vi "Func-엑셀 데이터를 그래프로 출력.vi"() -> ()   [LabVIEW 2015] (continued)
-10.012\n-18.3\t-18.31\t-10.011\n-18.3\t-18.31\t-10.009\n-18.3\t-18.31\t-10.008\n-18.3\t-18.31\t-10.009\n-18.3\t-18.31\t-10.009\n-18.3\t-18.31\t-10.008\n-18.3\t-18.31\t-10.003\n-18.3\t-18.31\t-10.002\n-18.3\t-18.31\t-10\n-18.3\t-18.31\t-10.001\n-18.3\t-18.31\t-10\n-18.3\t-18.31\t-9.994\n-18.3\t-18.31\t-9.993\n-18.3\t-18.31\t-9.993\n-18.3\t-18.31\t-9.993\n-18.3\t-18.31\t-9.989\n-18.3\t-18.31\t-9.99\n-18.3\t-18.31\t-9.995\n-18.3\t-18.31\t-9.995\n-18.3\t-18.31\t-9.993\n-18.3\t-18.31\t-9.99\n-18.3\t-18.31\t-9.987\n-18.3\t-18.31\t-9.984\n-18.3\t-18.31\t-9.979\n-18.3\t-18.31\t-9.975\n-18.3\t-18.31\t-9.972\n-18.3\t-18.31\t-9.973\n-18.3\t-18.31\t-9.969\n-18.3\t-18.31\t-9.965\n-18.3\t-18.31\t-9.962\n-18.3\t-18.31\t-9.963\n-18.3\t-18.31\t-9.964\n-18.3\t-18.31\t-9.962\n-18.3\t-18.31\t-9.967\n-18.3\t-18.31\t-9.969\n-18.3\t-18.31\t-9.97\n-18.3\t-18.31\t-9.971\n-18.3\t-18.31\t-9.968\n-18.3\t-18.31\t-9.967\n-18.3\t-18.31\t-9.961\n-18.3\t-18.31\t-9.957\n-18.3\t-18.31\t-9.955\n-18.3\t-18.31\t-9.948\n-18.3\t-18.31\t-9.948\n-18.3\t-18.31\t-9.945\n-18.3\t-18.31\t-9.948\n-18.3\t-18.31\t-9.948\n-18.3\t-18.31\t-9.948\n-18.3\t-18.31\t-9.95\n-18.3\t-18.31\t-9.949\n-18.3\t-18.31\t-9.947\n-18.3\t-18.31\t-9.941\n-18.3\t-18.31\t-9.941\n-18.3\t-18.31\t-9.939\n-18.3\t-18.31\t-9.937\n-18.3\t-18.31\t-9.936\n-18.3\t-18.31\t-9.938\n-18.3\t-18.31\t-9.933\n-18.3\t-18.31\t-9.931\n-18.3\t-18.31\t-9.929\n-18.3\t-18.31\t-9.925\n-18.3\t-18.31\t-9.925\n-18.3\t-18.31\t-9.925\n-18.3\t-18.31\t-9.927\n-18.3\t-18.31\t-9.927\n-18.3\t-18.31\t-9.93\n-18.3\t-18.31\t-9.926\n-18.3\t-18.31\t-9.923\n-18.3\t-18.31\t-9.92\n-18.3\t-18.31\t-9.916\n-18.3\t-18.31\t-9.915\n-18.3\t-18.31\t-9.911\n-18.3\t-18.31\t-9.911\n-18.3\t-18.31\t-9.911\n-18.3\t-18.31\t-9.91\n-18.3\t-18.31\t-9.911\n-18.3\t-18.31\t-9.912\n-18.3\t-18.31\t-9.911\n-18.3\t-18.31\t-9.911\n-18.3\t-18.31\t-9.908\n-18.3\t-18.31\t-9.909\n-18.3\t-18.31\t-9.905\n-18.3\t-18.31\t-9.902\n-18.3\t-18.31\t-9.899\n-18.3\t-18.31\t-9.898\n-18.3\t-18.31\t-9.895\n-18.3\t-18.31\t-9.894\n-18.3\t-18.31\t-9.895\n-18.3\t-18.31\t-9.891\n-18.3\t-18.31\t-9.886\n-18.3\t-18.31\t-9.886\n-18.3\t-18.31\t-9.885\n-18.3\t-18.31\t-9.882\n-18.3\t-18.31\t-9.877\n-18.3\t-18.31\t-9.878\n-18.3\t-18.31\t-9.88\n-18.3\t-18.31\t-9.879\n-18.3\t-18.31\t-9.879\n-18.3\t-18.31\t-9.879\n-18.3\t-18.31\t-9.879\n-18.3\t-18.31\t-9.875\n-18.3\t-18.31\t-9.875\n-18.3\t-18.31\t-9.875\n-18.3\t-18.31\t-9.873\n-18.3\t-18.31\t-9.87\n-18.3\t-18.31\t-9.868\n-18.3\t-18.31\t-9.868\n-18.3\t-18.31\t-9.867\n-18.3\t-18.31\t-9.865\n-18.3\t-18.31\t-9.864\n-18.3\t-18.31\t-9.864\n-18.3\t-18.31\t-9.866\n-18.3\t-18.31\t-9.865\n-18.3\t-18.31\t-9.863\n-18.3\t-18.31\t-9.861\n-18.3\t-18.31\t-9.861\n-18.3\t-18.31\t-9.866\n-18.3\t-18.31\t-9.861\n-18.3\t-18.31\t-9.861\n-18.3\t-18.31\t-9.86\n-18.3\t-18.31\t-9.856\n-18.3\t-18.31\t-9.852\n-18.3\t-18.31\t-9.849\n-18.3\t-18.31\t-9.847\n-18.3\t-18.31\t-9.844\n-18.3\t-18.31\t-9.842\n-18.3\t-18.31\t-9.844\n-18.3\t-18.31\t-9.846\n-18.3\t-18.31\t-9.841\n-18.3\t-18.31\t-9.84\n-18.3\t-18.31\t-9.84\n-18.3\t-18.31\t-9.841\n-18.3\t-18.31\t-9.837\n-18.3\t-18.31\t-9.835\n-18.3\t-18.31\t-9.836\n-18.3\t-18.31\t-9.834\n-18.3\t-18.31\t-9.834\n-18.3\t-18.31\t-9.832\n-18.3\t-18.31\t-9.832\n-18.3\t-18.31\t-9.832\n-18.3\t-18.31\t-9.83\n-18.3\t-18.31\t-9.833\n-18.3\t-18.31\t-9.83\n-18.3\t-18.31\t-9.827\n-18.3\t-18.31\t-9.824\n-18.3\t-18.31\t-9.823\n-18.3\t-18.31\t-9.823\n-18.3\t-18.31\t-9.82\n-18.3\t-18.31\t-9.82\n-18.3\t-18.31\t-9.821\n-18.3\t-18.31\t-9.82\n-18.3\t-18.31\t-9.821\n-18.3\t-18.31\t-9.821\n-18.3\t-18.31\t-9.821\n-18.3\t-18.31\t-9.822\n-18.3\t-18.31\t-9.82\n-18.3\t-18.31\t-9.817\n-18.3\t-18.31\t-9.815\n-18.3\t-18.31\t-9.812\n-18.3\t-18.31\t-9.807\n-18.3\t-18.31\t-9.801\n-18.3\t-18.31\t-9.803\n-18.3\t-18.31\t-9.802\n-18.3\t-18.31\t-9.802\n-18.3\t-18.31\t-9.801\n-18.3\t-18.31\t-9.8\n-18.3\t-18.31\t-9.799\n-18.3\t-18.31\t-9.799\n-18.3\t-18.31\t-9.797\n-18.3\t-18.31\t-9.797\n-18.3\t-18.31\t-9.795\n-18.3\t-18.31\t-9.795\n-18.3\t-18.31\t-9.793\n-18.3\t-18.31\t-9.788\n-18.3\t-18.31\t-9.79\n-18.3\t-18.31\t-9.788\n-18.3\t-18.31\t-9.789\n-18.3\t-18.31\t-9.785\n-18.3\t-18.31\t-9.787\n-18.3\t-18.31\t-9.786\n-18.3\t-18.31\t-9.784\n-18.3\t-18.31\t-9.782\n-18.3\t-18.31\t-9.782\n-18.3\t-18.31\t-9.782\n-18.3\t-18.31\t-9.783\n-18.3\t-18.31\t-9.783\n-18.3\t-18.31\t-9.774\n-18.3\t-18.31\t-9.775\n-18.3\t-18.31\t-9.77\n-18.3\t-18.31\t-9.769\n-18.3\t-18.31\t-9.768\n-18.3\t-18.31\t-9.769\n-18.3\t-18.31\t-9.778\n-18.3\t-18.31\t-9.775\n-18.3\t-18.31\t-9.779\n-18.3\t-18.31\t-9.777\n-18.3\t-18.31\t-9.777\n-18.3\t-18.31\t-9.778\n-18.3\t-18.31\t-9.77\n-18.3\t-18.31\t-9.767\n-18.3\t-18.31\t-9.765\n-18.3\t-18.31\t-9.76\n-18.3\t-18.31\t-9.755\n-18.3\t-18.31\t-9.75\n-18.3\t-18.31\t-9.749\n-18.3\t-18.31\t-9.749\n-18.3\t-18.31\t-9.748\n-18.3\t-18.31\t-9.751\n-18.3\t-18.31\t-9.752\n-18.3\t-18.31\t-9.754\n-18.3\t-18.31\t-9.752\n-18.3\t-18.31\t-9.752\n-18.3\t-18.31\t-9.748\n-18.3\t-18.31\t-9.745\n-18.3\t-18.31\t-9.743\n-18.3\t-18.31\t-9.739\n-18.3\t-18.31\t-9.74\n-18.3\t-18.31\t-9.74\n-18.3\t-18.31\t-9.74\n-18.3\t-18.31\t-9.735\n-18.3\t-18.31\t-9.735\n-18.3\t-18.31\t-9.736\n-18.3\t-18.31\t-9.734\n-18.3\t-18.31\t-9.73\n-18.3\t-18.31\t-9.732\n-18.3\t-18.31\t-9.736\n-18.3\t-18.31\t-9.733\n-18.3\t-18.31\t-9.732\n-18.3\t-18.31\t-9.729\n-18.3\t-18.31\t-9.729\n-18.3\t-18.31\t-9.725\n-18.3\t-18.31\t-9.72\n-18.3\t-18.31\t-9.721\n-18.3\t-18.31\t-9.72\n-18.3\t-18.31\t-9.722\n-18.3\t-18.31\t-9.722\n-18.3\t-18.31\t-9.721\n-18.3\t-18.31\t-9.722\n-18.3\t-18.31\t-9.721\n-18.3\t-18.31\t-9.721\n-18.3\t-18.31\t-9.718\n-18.3\t-18.31\t-9.719\n-18.3\t-18.31\t-9.718\n-18.3\t-18.31\t-9.719\n-18.3\t-18.31\t-9.721\n-18.3\t-18.31\t-9.719\n-18.3\t-18.31\t-9.716\n-18.3\t-18.31\t-9.711\n-18.3\t-18.31\t-9.712\n-18.3\t-18.31\t-9.712\n-18.3\t-18.31\t-9.707\n-18.3\t-18.31\t-9.708\n-18.3\t-18.31\t-9.71\n-18.3\t-18.31\t-9.709\n-18.3\t-18.31\t-9.705\n-18.3\t-18.31\t-9.704\n-18.3\t-18.31\t-9.702\n-18.3\t-18.31\t-9.7\n-18.3\t-18.31\t-9.7\n-18.3\t-18.31\t-9.702\n-18.3\t-18.31\t-9.704\n-18.3\t-18.31\t-9.701\n-18.3\t-18.31\t-9.702\n-18.3\t-18.31\t-9.699\n-18.3\t-18.31\t-9.698\n-18.3\t-18.31\t-9.695\n-18.3\t-18.31\t-9.695\n-18.3\t-18.31\t-9.695\n-18.3\t-18.31\t-9.694\n-18.3\t-18.31\t-9.695\n-18.3\t-18.31\t-9.691\n-18.3\t-18.31\t-9.689\n-18.3\t-18.31\t-9.686\n-18.3\t-18.31\t-9.684\n-18.3\t-18.31\t-9.68\n-18.3\t-18.31\t-9.678\n-18.3\t-18.31\t-9.679\n-18.3\t-18.31\t-9.68\n-18.3\t-18.31\t-9.68\n-18.3\t-18.31\t-9.678\n-18.3\t-18.31\t-9.68\n-18.3\t-18.31\t-9.679\n-18.3\t-18.31\t-9.677\n-18.3\t-18.31\t-9.675\n-18.3\t-18.31\t-9.673\n-18.3\t-18.31\t-9.674\n-18.3\t-18.31\t-9.675\n-18.3\t-18.31\t-9.674\n-18.3\t-18.31\t-9.672\n-18.3\t-18.31\t-9.67\n-18.3\t-18.31\t-9.67\n-18.3\t-18.31\t-9.669\n-18.3\t-18.31\t-9.666\n-18.3\t-18.31\t-9.667\n-18.3\t-18.31\t-9.666\n-18.3\t-18.31\t-9.666\n-18.3\t-18.31\t-9.664\n-18.3\t-18.31\t-9.663\n-18.3\t-18.31\t-9.663\n-18.3\t-18.31\t-9.663\n-18.3\t-18.31\t-9.661\n-18.3\t-18.31\t-9.656\n-18.3\t-18.31\t-9.654\n-18.3\t-18.31\t-9.654\n-18.3\t-18.31\t-9.654\n-18.3\t-18.31\t-9.652\n-18.3\t-18.31\t-9.65\n-18.3\t-18.31\t-9.652\n-18.3\t-18.31\t-9.654\n-18.3\t-18.31\t-9.65\n-18.3\t-18.31\t-9.647\n-18.3\t-18.31\t-9.644\n-18.3\t-18.31\t-9.646\n-18.3\t-18.31\t-9.646\n-18.3\t-18.31\t-9.642\n-18.3\t-18.31\t-9.645\n-18.3\t-18.31\t-9.643\n-18.3\t-18.31\t-9.645\n-18.3\t-18.31\t-9.639\n-18.3\t-18.31\t-9.639\n-18.3\t-18.31\t-9.639\n-18.3\t-18.31\t-9.639\n-18.3\t-18.31\t-9.641\n-18.3\t-18.31\t-9.637\n-18.3\t-18.31\t-9.639\n-18.3\t-18.31\t-9.639\n-18.3\t-18.31\t-9.637\n-18.3\t-18.31\t-9.629\n-18.3\t-18.31\t-9.624\n-18.3\t-18.31\t-9.622\n-18.3\t-18.31\t-9.62\n-18.3\t-18.31\t-9.619\n-18.3\t-18.31\t-9.62\n-18.3\t-18.31\t-9.62\n-18.3\t-18.31\t-9.62\n-18.3\t-18.31\t-9.621\n-18.3\t-18.31\t-9.624\n-18.3\t-18.31\t-9.625\n-18.3\t-18.31\t-9.622\n-18.3\t-18.31\t-9.625\n-18.3\t-18.31\t-9.624\n-18.3\t-18.31\t-9.621\n-18.3\t-18.31\t-9.619\n-18.3\t-18.31\t-9.613\n-18.3\t-18.31\t-9.609\n-18.3\t-18.31\t-9.607\n-18.3\t-18.31\t-9.607\n-18.3\t-18.31\t-9.605\n-18.3\t-18.31\t-9.609\n-18.3\t-18.31\t-9.613\n-18.3\t-18.31\t-9.613\n-18.3\t-18.31\t-9.614\n-18.3\t-18.31\t-9.613\n-18.3\t-18.31\t-9.611\n-18.3\t-18.31\t-9.607\n-18.3\t-18.31\t-9.604\n-18.3\t-18.31\t-9.604\n-18.3\t-18.31\t-9.601\n-18.3\t-18.31\t-9.6\n-18.3\t-18.31\t-9.602\n-18.3\t-18.31\t-9.604\n-18.3\t-18.31\t-9.603\n-18.3\t-18.31\t-9.602\n-18.3\t-18.31\t-9.603\n-18.3\t-18.31\t-9.606\n-18.3\t-18.31\t-9.604\n-18.3\t-18.31\t-9.6\n-18.3\t-18.31\t-9.602\n-18.3\t-18.31\t-9.6\n-18.3\t-18.31\t-9.601\n-18.3\t-18.31\t-9.598\n-18.3\t-18.31\t-9.598\n-18.3\t-18.31\t-9.595\n-18.3\t-18.31\t-9.593\n-18.3\t-18.31\t-9.594\n-18.3\t-18.31\t-9.594\n-18.3\t-18.31\t-9.595\n-18.3\t-18.31\t-9.592\n-18.3\t-18.31\t-9.598\n-18.3\t-18.31\t-9.596\n-18.3\t-18.31\t-9.594\n-18.3\t-18.31\t-9.588\n-18.3\t-18.31\t-9.587\n-18.3\t-18.31\t-9.585\n-18.3\t-18.31\t-9.579\n-18.3\t-18.31\t-9.579\n-18.3\t-18.31\t-9.574\n-18.3\t-18.31\t-9.578\n-18.3\t-18.31\t-9.575\n-18.3\t-18.31\t-9.575\n-18.3\t-18.31\t-9.575\n-18.3\t-18.31\t-9.573\n-18.227\t-18.25\t-9.109\n-18.143\t-18.18\t-9.102\n-18.06\t-18.12\t-9.09\n-17.977\t-18.32\t-9.09\n-17.893\t-18.38\t-9.096\n-17.81\t-18.43\t-9.092\n-17.727\t-18.51\t-9.087\n-17.643\t-18.57\t-9.085\n-17.56\t-18.62\t-9.089\n-17.477\t-18.68\t-9.081\n-17.393\t-18.74\t-9.075\n-17.31\t-18.79\t-9.079\n-17.227\t-18.83\t-9.069\n-17.143\t-18.86\t-9.073\n-17.06\t-18.88\t-9.07\n-16.977\t-18.89\t-9.072\n-16.893\t-18.87\t-9.071\n-16.81\t-18.86\t-9.067\n-16.727\t-18.84\t-9.071\n-16.643\t-18.82\t-9.076\n-16.56\t-18.78\t-9.072\n-16.477\t-18.73\t-9.069\n-16.393\t-18.67\t-9.07\n-16.31\t-18.62\t-9.075\n-16.227\t-18.55\t-9.071\n-16.143\t-18.48\t-9.073\n-16.06\t-18.41\t-9.074\n-15.977\t-18.34\t-9.069\n-15.893\t-18.27\t-9.074\n-15.81\t-18.18\t-9.077\n-15.727\t-18.1\t-9.073\n-15.643\t-18.01\t-9.086\n-15.56\t-17.91\t-9.08\n-15.477\t-17.82\t-9.078\n-15.393\t-17.73\t-9.079\n-15.31\t-17.63\t-9.077\n-15.227\t-17.55\t-9.076\n-15.143\t-17.46\t-9.087\n-15.06\t-17.36\t-9.075\n-14.977\t-17.27\t-9.072\n-14.893\t-17.17\t-9.07\n-14.81\t-17.08\t-9.071\n-14.727\t-16.99\t-9.069\n-14.643\t-16.9\t-9.069\n-14.56\t-16.81\t-9.06\n-14.477\t-16.73\t-9.06\n-14.393\t-16.65\t-9.052\n-14.31\t-16.57\t-9.044\n-14.227\t-16.48\t-9.036\n-14.143\t-16.4\t-9.035\n-14.06\t-16.31\t-9.027\n-13.977\t-16.23\t-9.016\n-13.893\t-16.16\t-9.013\n-13.81\t-16.07\t-9\n-13.727\t-15.99\t-8.993\n-13.643\t-15.92\t-8.982\n-13.56\t-15.85\t-8.973\n-13.477\t-15.77\t-8.961\n-13.393\t-15.69\t-8.946\n-13.31\t-15.61\t-8.935\n-13.227\t-15.53\t-8.924\n-13.143\t-15.45\t-8.911\n-13.06\t-15.38\t-8.898\n-12.977\t-15.3\t-8.889\n-12.893\t-15.23\t-8.865\n-12.81\t-15.14\t-8.849\n-12.727\t-15.08\t-8.828\n-12.643\t-15\t-8.819\n-12.56\t-14.92\t-8.789\n-12.477\t-14.84\t-8.776\n-12.393\t-14.76\t-8.756\n-12.31\t-14.68\t-8.729\n-12.227\t-14.61\t-8.712\n-12.143\t-14.54\t-8.686\n-12.06\t-14.46\t-8.679\n-11.977\t-14.39\t-8.652\n-11.893\t-14.31\t-8.623\n-11.81\t-14.24\t-8.606\n-11.727\t-14.15\t-8.582\n-11.643\t-14.07\t-8.555\n-11.56\t-13.99\t-8.529\n-11.477\t-13.91\t-8.505\n-11.393\t-13.83\t-8.469\n-11.31\t-13.75\t-8.455\n-11.227\t-13.67\t-8.418\n-11.143\t-13.59\t-8.395\n-11.06\t-13.51\t-8.368\n-10.977\t-13.43\t-8.341\n-10.893\t-13.35\t-8.308\n-10.81\t-13.27\t-8.281\n-10.727\t-13.19\t-8.244\n-10.643\t-13.11\t-8.217\n-10.56\t-13.04\t-8.188\n-10.477\t-12.96\t-8.153\n-10.393\t-12.89\t-8.131\n-10.31\t-12.81\t-8.098\n-10.227\t-12.74\t-8.061\n-10.143\t-12.66\t-8.029\n-10.06\t-12.6\t-8.002\n-9.977\t-12.52\t-7.962\n-9.893\t-12.44\t-7.935\n-9.81\t-12.36\t-7.898\n-9.727\t-12.28\t-7.868\n-9.643\t-12.21\t-7.835\n-9.56\t-12.12\t-7.791\n-9.477\t-12.05\t-7.763\n-9.393\t-11.96\t-7.726\n-9.31\t-11.88\t-7.688\n-9.227\t-11.8\t-7.656\n-9.143\t-11.74\t-7.614\n-9.06\t-11.65\t-7.577\n-8.977\t-11.57\t-7.539\n-8.893\t-11.5\t-7.497\n-8.81\t-11.42\t-7.463\n-8.727\t-11.34\t-7.415\n-8.643\t-11.26\t-7.379\n-8.56\t-11.19\t-7.333\n-8.477\t-11.11\t-7.288\n-8.393\t-11.03\t-7.259\n-8.31\t-10.94\t-7.211\n-8.227\t-10.86\t-7.166\n-8.143\t-10.78\t-7.121\n-8.06\t-10.7\t-7.076\n-7.977\t-10.62\t-7.039\n-7.893\t-10.53\t-6.994\n-7.81\t-10.45\t-6.95\n-7.727\t-10.37\t-6.907\n-7.643\t-10.28\t-6.863\n-7.56\t-10.2\t-6.817\n-7.477\t-10.12\t-6.769\n-7.393\t-10.03\t-6.723\n-7.31\t-9.95\t-6.679\n-7.227\t-9.87\t-6.632\n-7.143\t-9.79\t-6.595\n-7.06\t-9.72\t-6.54\n-6.977\t-9.65\t-6.496\n-6.893\t-9.57\t-6.446\n-6.81\t-9.5\t-6.399\n-6.727\t-9.41\t-6.343\n-6.643\t-9.34\t-6.3\n-6.56\t-9.26\t-6.254\n-6.477\t-9.18\t-6.203\n-6.393\t-9.1\t-6.157\n-6.31\t-9.03\t-6.098\n-6.227\t-8.95\t-6.05\n-6.143\t-8.87\t-6.001\n-6.06\t-8.79\t-5.95\n-5.977\t-8.71\t-5.889\n-5.893\t-8.63\t-5.837\n-5.81\t-8.55\t-5.788\n-5.727\t-8.48\t-5.736\n-5.643\t-8.4\t-5.683\n-5.56\t-8.32\t-5.622\n-5.477\t-8.24\t-5.575\n-5.393\t-8.17\t-5.516\n-5.31\t-8.08\t-5.458\n-5.227\t-8\t-5.407\n-5.143\t-7.92\t-5.352\n-5.06\t-7.84\t-5.297\n-4.977\t-7.76\t-5.236\n-4.893\t-7.69\t-5.187\n-4.81\t-7.6\t-5.127\n-4.727\t-7.53\t-5.066\n-4.643\t-7.45\t-5.014\n-4.56\t-7.36\t-4.957\n-4.477\t-7.28\t-4.905\n-4.393\t-7.21\t-4.846\n-4.31\t-7.13\t-4.779\n-4.227\t-7.04\t-4.722\n-4.143\t-6.96\t-4.671\n-4.06\t-6.87\t-4.606\n-3.977\t-6.79\t-4.545\n-3.893\t-6.71\t-4.485\n-3.81\t-6.64\t-4.427\n-3.727\t-6.56\t-4.373\n-3.643\t-6.47\t-4.308\n-3.56\t-6.4\t-4.246\n-3.477\t-6.32\t-4.18\n-3.393\t-6.24\t-4.129\n-3.31\t-6.17\t-4.067\n-3.227\t-6.08\t-4.008\n-3.143\t-6\t-3.941\n-3.06\t-5.92\t-3.88\n-2.977\t-5.84\t-3.825\n-2.893\t-5.76\t-3.755\n-2.81\t-5.69\t-3.699\n-2.727\t-5.6\t-3.637\n-2.643\t-5.52\t-3.577\n-2.56\t-5.44\t-3.504\n-2.477\t-5.36\t-3.445\n-2.393\t-5.28\t-3.382\n-2.31\t-5.2\t-3.318\n-2.227\t-5.12\t-3.262\n-2.143\t-5.05\t-3.192\n-2.06\t-4.97\t-3.136\n-1.977\t-4.89\t-3.071\n-1.893\t-4.81\t-3.002\n-1.81\t-4.72\t-2.941\n-1.727\t-4.63\t-2.881\n-1.643\t-4.55\t-2.809\n-1.56\t-4.46\t-2.746\n-1.477\t-4.39\t-2.687\n-1.393\t-4.31\t-2.615\n-1.31\t-4.22\t-2.555\n-1.227\t-4.14\t-2.477\n-1.143\t-4.06\t-2.428\n-1.06\t-3.99\t-2.352\n-0.977\t-3.9\t-2.289\n-0.893\t-3.8\t-2.217\n-0.81\t-3.72\t-2.159\n-0.727\t-3.64\t-2.092\n-0.643\t-3.56\t-2.022\n-0.56\t-3.48\t-1.96\n-0.477\t-3.41\t-1.9\n-0.393\t-3.32\t-1.831\n-0.31\t-3.25\t-1.765\n-0.227\t-3.17\t-1.698\n-0.143\t-3.09\t-1.629\n-0.06\t-3\t-1.562\n0.023\t-2.93\t-1.496\n0.107\t-2.85\t-1.419\n0.19\t-2.77\t-1.354\n0.273\t-2.7\t-1.29\n0.357\t-2.61\t-1.221\n0.44\t-2.53\t-1.153\n0.523\t-2.45\t-1.084\n0.607\t-2.37\t-1.016\n0.69\t-2.29\t-0.95\n0.773\t-2.22\t-0.875\n0.857\t-2.14\t-0.811\n0.94\t-2.06\t-0.741\n1.023\t-1.99\t-0.668\n1.107\t-1.91\t-0.607\n1.19\t-1.84\t-0.53\n1.273\t-1.75\t-0.467\n1.357\t-1.68\t-0.404\n1.44\t-1.59\t-0.325\n1.523\t-1.51\t-0.259\n1.607\t-1.44\t-0.194\n1.69\t-1.35\t-0.114\n1.773\t-1.27\t-0.052\n1.857\t-1.2\t0.02\n1.94\t-1.12\t0.099\n2.023\t-1.04\t0.156\n2.107\t-0.96\t0.223\n2.19\t-0.88\t0.305\n2.273\t-0.8\t0.365\n2.357\t-0.72\t0.436\n2.44\t-0.64\t0.509\n2.523\t-0.56\t0.589\n2.607\t-0.48\t0.65\n2.69\t-0.41\t0.719\n2.773\t-0.33\t0.798\n2.857\t-0.25\t0.863\n2.94\t-0.16\t0.939\n3.023\t-0.08\t1.005\n3.107\t0\t1.065\n3.19\t0.08\t1.145\n3.3\t0.14\t1.216\n3.3\t0.15\t1.219\n3.3\t0.16\t1.222\n3.3\t0.18\t1.229\n3.3\t0.18\t1.238\n3.3\t0.19\t1.246\n3.3\t0.2\t1.252\n3.3\t0.21\t1.26\n3.3\t0.22\t1.266\n3.3\t0.23\t1.275\n3.3\t0.23\t1.279\n3.3\t0.25\t1.286\n3.3\t0.25\t1.295\n3.3\t0.25\t1.304\n3.3\t0.26\t1.311\n3.3\t0.27\t1.316\n3.3\t0.28\t1.327\n3.3\t0.29\t1.33\n3.3\t0.29\t1.333\n3.3\t0.3\t1.335\n3.3\t0.31\t1.337\n3.3\t0.32\t1.343\n3.3\t0.33\t1.349\n3.3\t0.34\t1.358\n3.3\t0.35\t1.369\n3.3\t0.35\t1.378\n3.3\t0.36\t1.387\n3.3\t0.37\t1.401\n3.3\t0.38\t1.41\n3.3\t0.39\t1.414\n3.3\t0.4\t1.419\n3.3\t0.41\t1.425\n3.3\t0.42\t1.432\n3.3\t0.42\t1.437\n3.3\t0.43\t1.442\n3.3\t0.43\t1.451\n3.3\t0.44\t1.458\n3.3\t0.45\t1.466\n3.3\t0.46\t1.472\n3.3\t0.46\t1.478\n3.3\t0.47\t1.483\n3.3\t0.48\t1.489\n3.3\t0.49\t1.502\n3.3\t0.5\t1.509\n3.3\t0.51\t1.518\n3.3\t0.51\t1.531\n3.3\t0.51\t1.538\n3.3\t0.52\t1.546\n3.3\t0.53\t1.554\n3.3\t0.53\t1.562\n3.3\t0.54\t1.568\n3.3\t0.55\t1.571\n3.3\t0.56\t1.579\n3.3\t0.57\t1.586\n3.3\t0.57\t1.589\n3.3\t0.58\t1.595\n3.3\t0.59\t1.602\n3.3\t0.59\t1.614\n3.3\t0.6\t1.621\n3.3\t0.6\t1.626\n3.3\t0.61\t1.635\n3.3\t0.62\t1.642\n3.3\t0.63\t1.645\n3.3\t0.63\t1.654\n3.3\t0.64\t1.658\n3.3\t0.65\t1.665\n3.3\t0.65\t1.673\n3.3\t0.66\t1.679\n3.3\t0.67\t1.686\n3.3\t0.68\t1.695\n3.3\t0.68\t1.704\n3.3\t0.69\t1.709\n3.3\t0.7\t1.719\n3.3\t0.71\t1.727\n3.3\t0.72\t1.732\n3.3\t0.72\t1.741\n3.3\t0.73\t1.743\n3.3\t0.73\t1.751\n3.3\t0.74\t1.762\n3.3\t0.75\t1.765\n3.3\t0.76\t1.775\n3.3\t0.77\t1.785\n3.3\t0.77\t1.795\n3.3\t0.78\t1.8\n3.3\t0.79\t1.807\n3.3\t0.8\t1.817\n3.3\t0.81\t1.82\n3.3\t0.82\t1.832\n3.3\t0.82\t1.837\n3.3\t0.83\t1.845\n3.3\t0.84\t1.858\n3.3\t0.85\t1.861\n3.3\t0.85\t1.869\n3.3\t0.86\t1.875\n3.3\t0.87\t1.88\n3.3\t0.88\t1.884\n3.3\t0.89\t1.891\n3.3\t0.9\t1.898\n3.3\t0.91\t1.903\n3.3\t0.92\t1.91\n3.3\t0.93\t1.918\n3.3\t0.93\t1.923\n3.3\t0.93\t1.929\n3.3\t0.94\t1.938\n3.3\t0.95\t1.947\n3.3\t0.96\t1.956\n3.3\t0.96\t1.96\n3.3\t0.97\t1.967\n3.3\t0.98\t1.979\n3.3\t0.99\t1.98\n3.3\t1\t1.987\n3.3\t1.01\t1.992\n3.3\t1.02\t2.002\n3.3\t1.02\t2.011\n3.3\t1.03\t2.016\n3.3\t1.04\t2.025\n3.3\t1.05\t2.032\n3.3\t1.06\t2.041\n3.3\t1.07\t2.048\n3.3\t1.08\t2.058\n3.3\t1.09\t2.064\n3.3\t1.1\t2.07\n3.3\t1.1\t2.078\n3.3\t1.11\t2.085\n3.3\t1.12\t2.089\n3.3\t1.13\t2.103\n3.3\t1.14\t2.109\n3.3\t1.15\t2.116\n3.3\t1.16\t2.125\n3.3\t1.17\t2.132\n3.3\t1.18\t2.14\n3.3\t1.18\t2.144\n3.3\t1.19\t2.151\n3.3\t1.2\t2.157\n3.3\t1.21\t2.164\n3.3\t1.21\t2.171\n3.3\t1.22\t2.174\n3.3\t1.23\t2.183\n3.3\t1.24\t2.186\n3.3\t1.25\t2.192\n3.3\t1.26\t2.202\n3.3\t1.27\t2.207\n3.3\t1.27\t2.215\n3.3\t1.28\t2.223\n3.3\t1.3\t2.23\n3.3\t1.3\t2.237\n3.3\t1.31\t2.244\n3.3\t1.32\t2.253\n3.3\t1.34\t2.262\n3.3\t1.34\t2.268\n3.3\t1.35\t2.274\n3.3\t1.35\t2.28\n3.3\t1.36\t2.29\n3.3\t1.37\t2.296\n3.3\t1.38\t2.301\n3.3\t1.39\t2.312\n3.3\t1.39\t2.32\n3.3\t1.4\t2.327\n3.3\t1.41\t2.338\n3.3\t1.42\t2.341\n3.3\t1.43\t2.348\n3.3\t1.43\t2.354\n3.3\t1.44\t2.36\n3.3\t1.45\t2.367\n3.3\t1.47\t2.375\n3.3\t1.48\t2.384\n3.3\t1.48\t2.39\n3.3\t1.49\t2.403\n3.3\t1.5\t2.405\n3.3\t1.51\t2.415\n3.3\t1.52\t2.421\n3.3\t1.52\t2.427\n3.3\t1.53\t2.433\n3.3\t1.54\t2.44\n3.3\t1.55\t2.45\n3.3\t1.56\t2.454\n3.3\t1.57\t2.462\n3.3\t1.58\t2.469\n3.3\t1.59\t2.478\n3.3\t1.6\t2.487\n3.3\t1.6\t2.493\n3.3\t1.6\t2.499\n3.3\t1.62\t2.508\n3.3\t1.62\t2.511\n3.3\t1.63\t2.518\n3.3\t1.64\t2.526\n3.3\t1.66\t2.532\n3.3\t1.67\t2.544\n3.3\t1.68\t2.553\n3.3\t1.69\t2.56\n3.3\t1.69\t2.571\n3.3\t1.7\t2.577\n3.3\t1.71\t2.582\n3.3\t1.72\t2.59\n3.3\t1.73\t2.594\n3.3\t1.74\t2.597\n3.3\t1.74\t2.603\n3.3\t1.75\t2.611\n3.3\t1.77\t2.618\n3.3\t1.77\t2.625\n3.3\t1.78\t2.631\n3.3\t1.79\t2.639\n3.3\t1.8\t2.646\n3.3\t1.81\t2.656\n3.3\t1.82\t2.664\n3.3\t1.83\t2.668\n3.3\t1.84\t2.679\n3.3\t1.85\t2.688\n3.3\t1.85\t2.696\n3.3\t1.86\t2.704\n3.3\t1.87\t2.709\n3.3\t1.88\t2.719\n3.3\t1.89\t2.729\n3.3\t1.9\t2.734\n3.3\t1.91\t2.741\n3.3\t1.92\t2.748\n3.3\t1.93\t2.756\n3.3\t1.94\t2.761\n3.3\t1.94\t2.768\n3.3\t1.95\t2.775\n3.3\t1.95\t2.782\n3.3\t1.96\t2.789\n3.3\t1.97\t2.795\n3.3\t1.98\t2.802\n3.3\t1.99\t2.809\n3.3\t2\t2.814\n3.3\t2.01\t2.82\n3.3\t2.02\t2.829\n3.3\t2.02\t2.835\n3.3\t2.03\t2.85\n3.3\t2.04\t2.856\n3.3\t2.05\t2.865\n3.3\t2.06\t2.87\n3.3\t2.07\t2.882\n3.3\t2.08\t2.888\n3.3\t2.09\t2.892\n3.3\t2.1\t2.897\n3.3\t2.1\t2.903\n3.3\t2.11\t2.913\n3.3\t2.12\t2.919\n3.3\t2.13\t2.927\n3.3\t2.14\t2.937\n3.3\t2.15\t2.944\n3.3\t2.15\t2.95\n3.3\t2.16\t2.957\n3.3\t2.17\t2.96\n3.3\t2.18\t2.97\n3.3\t2.18\t2.98\n3.3\t2.19\t2.986\n3.3\t2.19\t2.993\n3.3\t2.19\t3.003\n3.3\t2.2\t3.009\n3.3\t2.21\t3.014\n3.3\t2.22\t3.021\n3.3\t2.23\t3.03\n3.3\t2.23\t3.034\n3.3\t2.24\t3.042\n3.3\t2.25\t3.052\n3.3\t2.26\t3.062\n3.3\t2.26\t3.068\n3.3\t2.27\t3.072\n3.3\t2.27\t3.082\n3.3\t2.28\t3.091\n3.3\t2.29\t3.093\n3.3\t2.3\t3.098\n3.3\t2.3\t3.111\n3.3\t2.31\t3.121\n3.3\t2.33\t3.125\n3.3\t2.34\t3.135\n3.3\t2.35\t3.146\n3.3\t2.36\t3.154\n3.3\t2.36\t3.16\n3.3\t2.36\t3.167\n3.3\t2.37\t3.175\n3.3\t2.38\t3.18\n3.3\t2.39\t3.183\n3.3\t2.4\t3.185\n3.3\t2.4\t3.195\n3.3\t2.41\t3.201\n3.3\t2.42\t3.206\n3.3\t2.43\t3.217\n3.3\t2.44\t3.225\n3.3\t2.44\t3.231\n3.3\t2.44\t3.238\n3.3\t2.45\t3.243\n3.3\t
